vi "Get PID String.vi"(1 "PID Loop ID":string, 2 "PID Parameter":T1) -> (0 "Parameter String":string)   [LabVIEW 2014, in "PID Loop.lvclass"]
uses:
  PID Loop.lvclass
  String Parameters.ctl
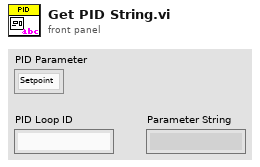
[diagram p1: front panel]
types:
  T1 = typedef "PID Loop.lvclass/String Parameters.ctl" = enum16{"Setpoint", "Process Variable", "Output", "Proportional Gain", "Integral Time", "Derivative Time", "Range High", "Range Low"}
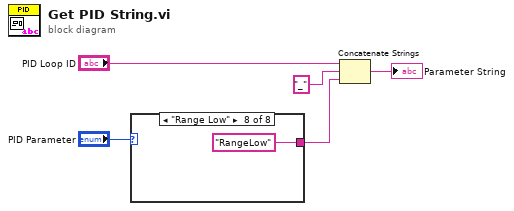
[diagram p0: block diagram]
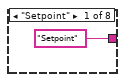
[diagram p2: hidden frame]
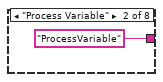
[diagram p3: hidden frame]
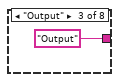
[diagram p4: hidden frame]
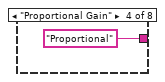
[diagram p5: hidden frame]
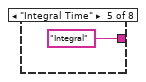
[diagram p6: hidden frame]
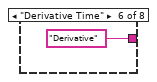
[diagram p7: hidden frame]
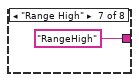
[diagram p8: hidden frame]
diagram:
  n1 = case shown="\"Range Low\"" "PID Parameter" {
    tunnel: ["Setpoint" "ProcessVariable" "Output" "Proportional" "Integral" "Derivative" "RangeHigh" "RangeLow"] -> w3
    frame "Setpoint" {
    }
    frame "Process Variable" {
    }
    frame "Output" {
    }
    frame "Proportional Gain" {
    }
    frame "Integral Time" {
    }
    frame "Derivative Time" {
    }
    frame "Range High" {
    }
    frame "Range Low" {
    }
  }
  n2 = Concatenate Strings("PID Loop ID", "_" ("string"), w3) -> (→"Parameter String":string)
